vi "CC FITS Calculate RA and DEC for Detector.vi"(8 "DEC":dbl, 9 "RA":dbl, 10 "ROT":dbl, 11 "Detector #":u16) -> (2 "DEC out":dbl, 3 "RA out":dbl)   [LabVIEW 2021]
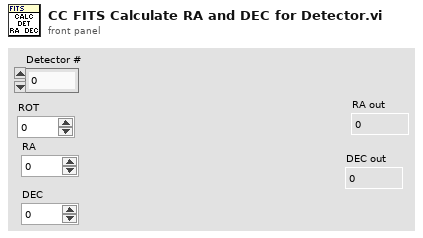
[diagram p1: front panel]
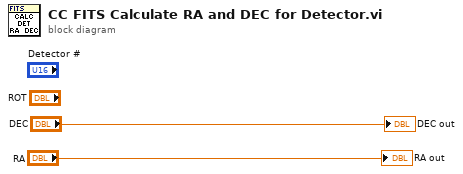
[diagram p0: block diagram]
diagram:
  "DEC out" <- "DEC"
  "RA out" <- "RA"
